vi "3458A Close Virtual Channels.vi"(8 "error in":errorcluster, 10 "Reset to preset mode (True)":bool=TRUE, 11 "session in":T1={"channels"=[], "sync unit"={"VISA"="", "type"=enum."Picotest U6200A"}, "awg unit"={"type"=enum."Agilent 331xxA to 332xxA", "VISA"="", "enable 10MHz ref"=FALSE, "cmi ckd2"={"VISA"="", "clock source"=enum."Auto", "manual ref clk"=FALSE, "ref clock [Hz]"=0.0}}, "sync mode"=enum."MASTER-SLAVE, MASTER clocked by TIMER", "streaming mode"=FALSE, "idn mode"=enum."Auto", "sampling mode"=enum."DCV", "Ts [s]"=0.0, "sample memory [B]"=0, "proc setup"={"channel id"=0, "packet size [smpl]"=0, "current timeout [s]"=0.0, "blk2blk timeout [s]"=0.0, "event time"=timestamp(0 s since 1904-01-01), "stop notifier"=refnum, "data queues"=[], "proc refs"=[], "bus semaphore"=refnum}, "sample size [B]"=0, "sample count"=0, "aux data"={"channel id"=0, "valid?"=[], "gain [V]"=[], "timestamp [s]"=[], "Ts [s]"=0.0, "abs timestamp"=timestamp(0 s since 1904-01-01), "t [deg C]"=[], "multiplex timestamp [s]"=-1.0, "only multiplex?"=FALSE, "multiplex smpl offset"=0, "overflow?"=FALSE}, "ranges [V]"=[], "aperture [s]"=0.0, "LEVEL trigger"={"edge"=enum."POS", "level [V]"=0.0, "coupling"=enum."DC"}, "trigger mode"=enum."AUTO", "measure temp.?"=FALSE, "disp mesages"=[], "shared bus?"=FALSE, "disable display?"=FALSE, "aper mode"=enum."Manual", "aper rules"=[], "multiplex"={"cycles"=0, "delay [s]"=0.0, "enabled"=FALSE, "overhead [s]"=1.0, "tot smpls"=0, "sub-rec"=0, "overhead [%]"=0.0}, "F8588 lpf"=enum."Off", "F8588 pll"=enum."Off", "F8588 couple"=enum."DC, auto"} {"channels"."Range [Vpk]" min=0.0}) -> (0 "error out":errorcluster, 3 "session out":T1={"channels"=[], "sync unit"={"VISA"="", "type"=enum."Picotest U6200A"}, "awg unit"={"type"=enum."Agilent 331xxA to 332xxA", "VISA"="", "enable 10MHz ref"=FALSE, "cmi ckd2"={"VISA"="", "clock source"=enum."Auto", "manual ref clk"=FALSE, "ref clock [Hz]"=0.0}}, "sync mode"=enum."MASTER-SLAVE, MASTER clocked by TIMER", "streaming mode"=FALSE, "idn mode"=enum."Auto", "sampling mode"=enum."DCV", "Ts [s]"=0.0, "sample memory [B]"=0, "proc setup"={"channel id"=0, "packet size [smpl]"=0, "current timeout [s]"=0.0, "blk2blk timeout [s]"=0.0, "event time"=timestamp(0 s since 1904-01-01), "stop notifier"=refnum, "data queues"=[], "proc refs"=[], "bus semaphore"=refnum}, "sample size [B]"=0, "sample count"=0, "aux data"={"channel id"=0, "valid?"=[], "gain [V]"=[], "timestamp [s]"=[], "Ts [s]"=0.0, "abs timestamp"=timestamp(0 s since 1904-01-01), "t [deg C]"=[], "multiplex timestamp [s]"=-1.0, "only multiplex?"=FALSE, "multiplex smpl offset"=0, "overflow?"=FALSE}, "ranges [V]"=[], "aperture [s]"=0.0, "LEVEL trigger"={"edge"=enum."POS", "level [V]"=0.0, "coupling"=enum."DC"}, "trigger mode"=enum."AUTO", "measure temp.?"=FALSE, "disp mesages"=[], "shared bus?"=FALSE, "disable display?"=FALSE, "aper mode"=enum."Manual", "aper rules"=[], "multiplex"={"cycles"=0, "delay [s]"=0.0, "enabled"=FALSE, "overhead [s]"=1.0, "tot smpls"=0, "sub-rec"=0, "overhead [%]"=0.0}, "F8588 lpf"=enum."Off", "F8588 pll"=enum."Off", "F8588 couple"=enum."DC, auto"} {"channels"."Range [Vpk]" min=0.0})   [LabVIEW 2020, in "3458A Virtual Digitizer.lvlib"]
doc: "Call this to close all instruments related to the opened session. It automatically does cleanup of digitizing processes, i.e. stops them, destroys data queues and notifiers."
uses:
  3458A Virtual Digitizer.lvlib
  3458A Digitizer Session.ctl
  3458A Virtual Channel Config.ctl
  Counter/Counter Session.ctl
  Counter/Counter Type.ctl
  AWG/AWG Session.ctl
  AWG/AWG Type.ctl
  AWG/CMI Clock Divider v2/CMI ckd2 Session.ctl
  AWG/CMI Clock Divider v2/CMI ckd2 Source Mode.ctl
  3458A Sync Mode.ctl
  3458A Idn Mode.ctl
  3458A Digitizing Low Levels/Configure/Sampling Mode.ctl
  3458A Digitizing Process Options.ctl
  3458A Data Packet.ctl
  3458A Aux Record Data.ctl
  3458A Digitizing Low Levels/Configure/Level Setup.ctl
  3458A Digitizing Low Levels/Configure/First Sample Trigger.ctl
  3458A Aperture Selection Mode.ctl
  3458A Multiplexing Config.ctl
  Fluke 8588A/F8588A Low Pass Filter.ctl
  Fluke 8588A/F8588A Phase Lock.ctl
  Fluke 8588A/F8588A Coupling.ctl
  3458A Digitizing Low Levels/3458A Digitizing Low Levels.lvlib
  AWG/AWG.lvlib
  Counter/Counter.lvlib
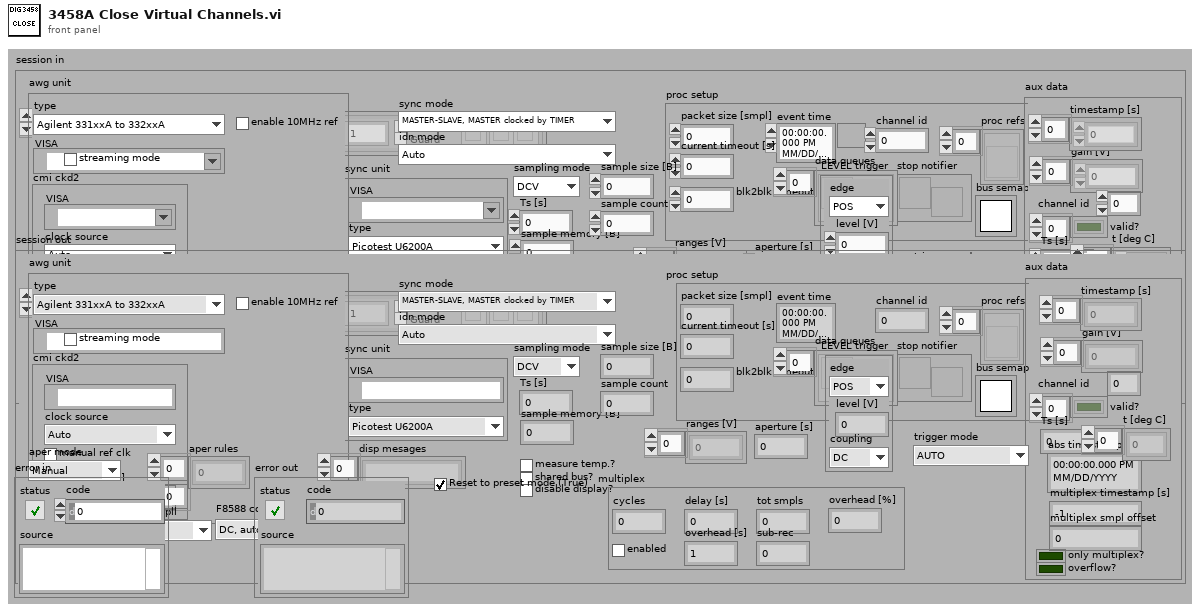
[diagram p1: front panel]
types:
  T1 = typedef "3458A Virtual Digitizer.lvlib/3458A Digitizer Session.ctl" = cluster{"channels":T2[], "sync unit":T3, "awg unit":T5, "sync mode":T9, "streaming mode":bool, "idn mode":T10, "sampling mode":T11, "Ts [s]":dbl, "sample memory [B]":i32, "proc setup":T12, "sample size [B]":i32, "sample count":i32, "aux data":T14, "ranges [V]":dbl[], "aperture [s]":dbl, "LEVEL trigger":T15, "trigger mode":T16, "measure temp.?":bool, "disp mesages":string[], "shared bus?":bool, "disable display?":bool, "aper mode":T17, "aper rules":dbl[][], "multiplex":T18, "F8588 lpf":T19, "F8588 pll":T20, "F8588 couple":T21}
  T2 = typedef "3458A Virtual Digitizer.lvlib/3458A Virtual Channel Config.ctl" = cluster{"VISA":refnum<visa-resource-name>, "Range [Vpk]":dbl, "btn clr":bool, "btn up":bool, "btn down":bool, "F8588":bool, "F8588 guard":bool}
  T3 = typedef "Counter.lvlib/Counter Session.ctl" = cluster{"VISA":refnum<visa-resource-name>, "type":T4}
  T4 = typedef "Counter.lvlib/Counter Type.ctl" = enum16{"Picotest U6200A", "dummy"}
  T5 = typedef "AWG.lvlib/AWG Session.ctl" = cluster{"type":T6, "VISA":refnum<visa-resource-name>, "enable 10MHz ref":bool, "cmi ckd2":T7}
  T6 = typedef "AWG.lvlib/AWG Type.ctl" = enum16{"Agilent 331xxA to 332xxA", "Agilent 335xxA to 336xxA", "Tektronix AFG3101C", "CMI Clock Divider v2", "dummy"}
  T7 = typedef "AWG.lvlib/CMI ckd2 Session.ctl" = cluster{"VISA":refnum<visa-resource-name>, "clock source":T8, "manual ref clk":bool, "ref clock [Hz]":dbl}
  T8 = typedef "AWG.lvlib/CMI ckd2 Source Mode.ctl" = enum16{"Auto", "LF clock", "HF clock", "Internal"}
  T9 = typedef "3458A Virtual Digitizer.lvlib/3458A Sync Mode.ctl" = enum16{"MASTER-SLAVE, MASTER clocked by TIMER", "MASTER-SLAVE, MASTER clocked by AWG", "ALL clocked by AWG", "MASTER-SLAVE, ALL clocked by TIMER", "ALL clocked by AWG with DFLL"}
  T10 = typedef "3458A Virtual Digitizer.lvlib/3458A Idn Mode.ctl" = enum16{"Auto", "Sequential (chn A, chn B, ...)", "From calibration string"}
  T11 = typedef "3458A Virtual Digitizer.lvlib/3458A Digitizing Low Levels.lvlib/Sampling Mode.ctl" = enum16{"DCV", "DSDC", "DSAC"}
  T12 = typedef "3458A Virtual Digitizer.lvlib/3458A Digitizing Process Options.ctl" = cluster{"channel id":i32, "packet size [smpl]":i32, "current timeout [s]":dbl, "blk2blk timeout [s]":dbl, "event time":timestamp, "stop notifier":refnum<notifier>, "data queues":refnum<queue>[], "proc refs":refnum<vi>[], "bus semaphore":T13}
  T13 = typedef "Semaphore RefNum" = refnum<k1>
  T14 = typedef "3458A Virtual Digitizer.lvlib/3458A Aux Record Data.ctl" = cluster{"channel id":i32, "valid?":bool[], "gain [V]":dbl[], "timestamp [s]":dbl[], "Ts [s]":dbl, "abs timestamp":timestamp, "t [deg C]":dbl[], "multiplex timestamp [s]":dbl, "only multiplex?":bool, "multiplex smpl offset":i64, "overflow?":bool}
  T15 = typedef "3458A Virtual Digitizer.lvlib/3458A Digitizing Low Levels.lvlib/Level Setup.ctl" = cluster{"edge":enum16{"POS", "NEG"}, "level [V]":dbl, "coupling":enum16{"DC", "AC"}}
  T16 = typedef "3458A Virtual Digitizer.lvlib/3458A Digitizing Low Levels.lvlib/First Sample Trigger.ctl" = enum16{"AUTO", "EXT", "SYN", "SGL", "HOLD", "LEVEL"}
  T17 = typedef "3458A Virtual Digitizer.lvlib/3458A Aperture Selection Mode.ctl" = enum16{"Manual", "Maximum", "Table"}
  T18 = typedef "3458A Multiplexing Config.ctl" = cluster{"cycles":i32, "delay [s]":dbl, "enabled":bool, "overhead [s]":dbl, "tot smpls":i64, "sub-rec":i32, "overhead [%]":dbl}
  T19 = typedef "F8588A Low Pass Filter.ctl" = enum16{"Off", "100 kHz", "3 MHz"}
  T20 = typedef "F8588A Phase Lock.ctl" = enum16{"Off", "1 MHz", "10 MHz"}
  T21 = typedef "F8588A Coupling.ctl" = enum16{"AC, 1 MOhm", "AC, 10 MOhm", "DC, 1 MOhm", "DC, 10 MOhm", "DC, auto"}
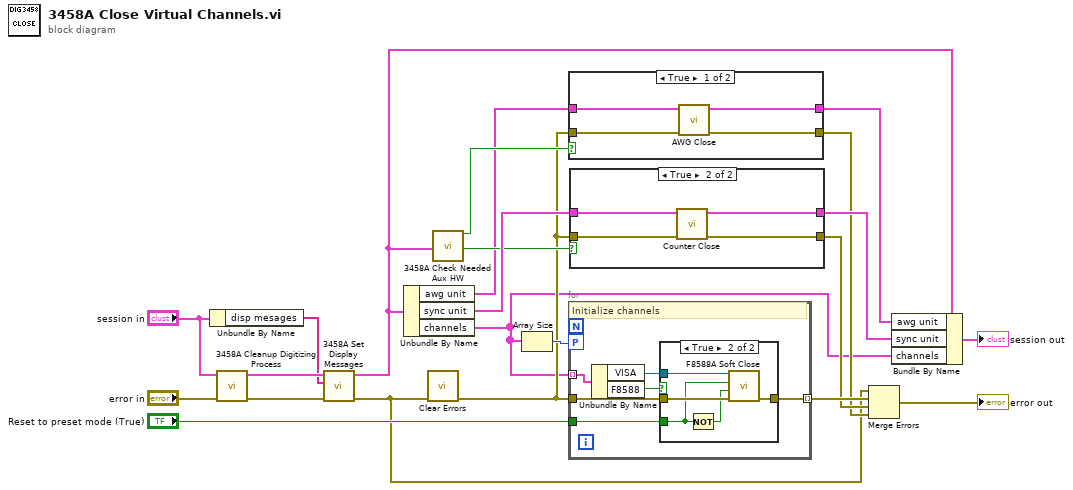
[diagram p0: block diagram]
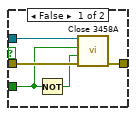
[diagram p4: hidden frame]
diagram:
  n1 = Unbundle By Name("session in") -> ("disp mesages"=w2:string[])
  n2 = call "3458A Cleanup Digitizing Process.vi"("error in"="error in", "session in"="session in") -> ("error out"=w7:errorcluster, "session out"=w5:T1)  [unwired: 8 in]
  n3 = call "3458A Set Display Messages.vi"("error in (no error)"=w7, "display strings"=w2, "digitizer session in"=w5) -> ("error out"=w6:errorcluster, "digitizer session out"=w4:T1)  [unwired: 7 in]
  n4 = Unbundle By Name(w4) -> ("awg unit"=w9:T5, "sync unit"=w20:T3, "channels"=w1:T2[])
  n5 = call <vilib>:"Clear Errors.vi"("error in (no error)"=w6) -> ("error out"=w8:errorcluster)  [unwired: 5 in, 1 out]
  n6 = call "3458A Check Needed Aux HW.vi"("digitizer session"=w4) -> ("uses AWG clocking?"=w12:bool, "uses counter?"=w13:bool)  [unwired: 13 in, 4 out]
  n7 = Array Size(array=w1) -> (size(s)=w22:i32)
  n8 = case shown="True" w12 {
    tunnel: w8 -> [w26 w28]
    tunnel: [w23 w28] -> w11
    tunnel: w9 -> [w25 w27]
    tunnel: [w24 w27] -> w10
    frame True {
      # "Initialize AWG"
      n9 = call "AWG Close.vi"("error in (no error)"=w26, "awg session in"=w25) -> ("error out"=w23:errorcluster, "awg session out"=w24:T5)  [unwired: 8 in]
    }
    frame False {
    }
  }
  n10 = for {
    tunnel: w8 -> [w34]
    tunnel: w1 -> [w31] mode=indexing
    workers-P: w22 -> [_]
    tunnel: [w33] -> w21 mode=indexing
    tunnel: "Reset to preset mode (True)" -> [w30]
    # "Initialize channels"
    n11 = Unbundle By Name(w31) -> ("VISA"=w32:refnum<visa-resource-name>, "F8588"=w29:bool)
    n12 = case shown="True" w29 {
      tunnel: w34 -> [w39 w44]
      tunnel: [w38 w43] -> w33
      tunnel: w32 -> [w37 w42]
      tunnel: w30 -> [w35 w40]
      frame False {
        n13 = Not(x=w35) -> (.not. x?=w36:bool)
        n14 = call "Close 3458A.vi"("error in (no error)"=w39, "keep display in whatever mode? (False)"=w36, "Reset to preset mode (True)"=w35, "VISA resource name"=w37) -> ("error out"=w38:errorcluster)  [unwired: 7 in]
      }
      frame True {
        n15 = Not(x=w40) -> (.not. x?=w41:bool)
        n16 = call "F8588A Soft Close.vi"("error in (no error)"=w44, "keep display in whatever mode? (False)"=w41, "Reset to preset mode (True)"=w40, "VISA resource name"=w42) -> ("error out"=w43:errorcluster)  [unwired: 7 in]
      }
    }
  }
  n17 = case shown="True" w13 {
    tunnel: w8 -> [w45 w50]
    tunnel: w20 -> [w46 w49]
    tunnel: [w45 w47] -> w18
    tunnel: [w46 w48] -> w19
    frame False {
      # "Initialize AWG"
    }
    frame True {
      # "Initialize counter"
      n18 = call "Counter Close.vi"("error in"=w50, "couner session in"=w49) -> ("error out"=w47:errorcluster, "counter session out"=w48:T3)  [unwired: 8 in]
    }
  }
  n19 = Merge Errors(w6, w21, w18, w11) -> (→"error out":errorcluster)
  n20 = Bundle By Name(cluster=w4, "awg unit"=w10, "sync unit"=w19, "channels"=w1) -> (→"session out":T1)
